vi "ZMQ queue reads.vi"(0 "context in":refnum<class "zmq_context.lvclass">, 1 "Current ZMQ Log":refnum<vi>, 5 "zmq_socket in":refnum<class "zmq_socket.lvclass">, 7 "queue in":refnum<queue>, 9 "Stop":refnum<vi>, 11 "Error in":errorcluster) -> (6 "queue out":refnum<queue>, 10 "ZMQ error out":errorcluster, 15 "Queue error out":errorcluster)   [LabVIEW 2018]
uses:
  <vilib>/addons/zeromq/zmq_socket.lvclass
  Event Sources.ctl
  <vilib>/addons/zeromq/zmq_context.lvclass
  <vilib>/Platform/TimedLoop/XDataNode/timing_clust.ctl
  <vilib>/Platform/TimedLoop/XDataNode/nitl_modes.ctl
  <vilib>/Platform/TimedLoop/XDataNode/wakeup.ctl
  <vilib>/addons/zeromq/poll_type.ctl
  <vilib>/Utility/file.llb/Write Delimited Spreadsheet (string).vi
  <vilib>/addons/zeromq/zmq_poll_scalar.vi
  <vilib>/platform/TimedLoop/XDataNode/XDataNode.xnode
  <vilib>/regexp/Match Regular Expression.xnode
  <vilib>/addons/zeromq/zeromq.lvlib
  <vilib>/Platform/TimedLoop/XDataNode/XDNodeRunTimeDep.lvlib
panel:
  in  "Stop":bool
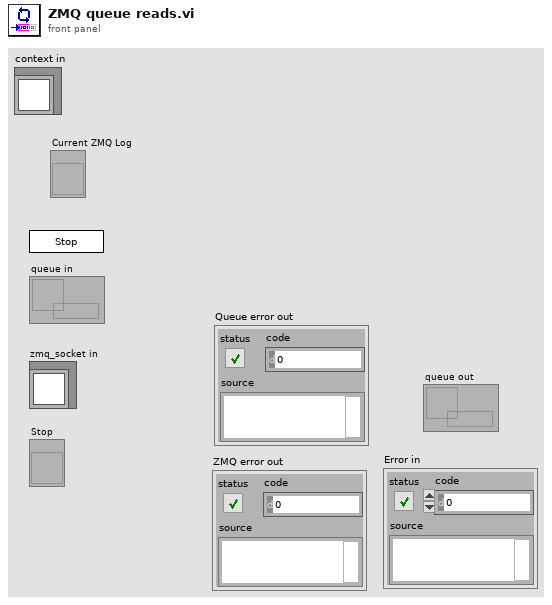
[diagram p1: front panel]
types:
  T1 = typedef "Event Sources.ctl" = enum16{"ZMQ", "INTERNAL", "Check_Errors", "Send_ZMQ_Reply", "Save_PMT_Voltages", "Set_Ramp_Voltage", "Restore PMT Voltages"}
  T2 = typedef "XDNodeRunTimeDep.lvlib/timing_clust.ctl" = cluster{"Expected End [f-1]":u64, "Actual End [f-1]":u64, "Finished Late? [f-1]":bool, "Expected End [i-1]":u64, "Actual End [i-1]":u64, "Finished Late? [i-1]":bool, "Expected Start [i]":u64, "Actual Start [i]":u64, "Expected Start [f]":u64, "Actual Start [f]":u64, "Source Name":string, "Structure Name":string, "Period":i64, "Deadline":i64, "Offset":i64, "Start":i64, "Priority":i32, "Timeout":i32, "Mode":T3, "Wakeup Reason":T4, "Error":errorcluster, "Source Type":string, "Secondary Source Type":string, "Global End Time":u64, "Global Start Time":u64, "Frame Duration":u64, "Iteration Duration":u64, "Assigned CPU":i32, "I/O Scan Engine Mode":u32}
  T3 = typedef "XDNodeRunTimeDep.lvlib/nitl_modes.ctl" = enum32{"No Change", "Process missed periods, maintain original phase", "Discard missed periods, maintain original phase", "Process missed periods, ignore original phase", "Discard missed periods, ignore original phase"}
  T4 = typedef "XDNodeRunTimeDep.lvlib/wakeup.ctl" = enum32{"Normal", "Aborted", "Asynchronous wakeup", "Timing source error", "Timed loop error", "Timeout"}
  T5 = typedef "zeromq.lvlib/poll_type.ctl" = enum16{"None", "In", "Out", "In/Out"}
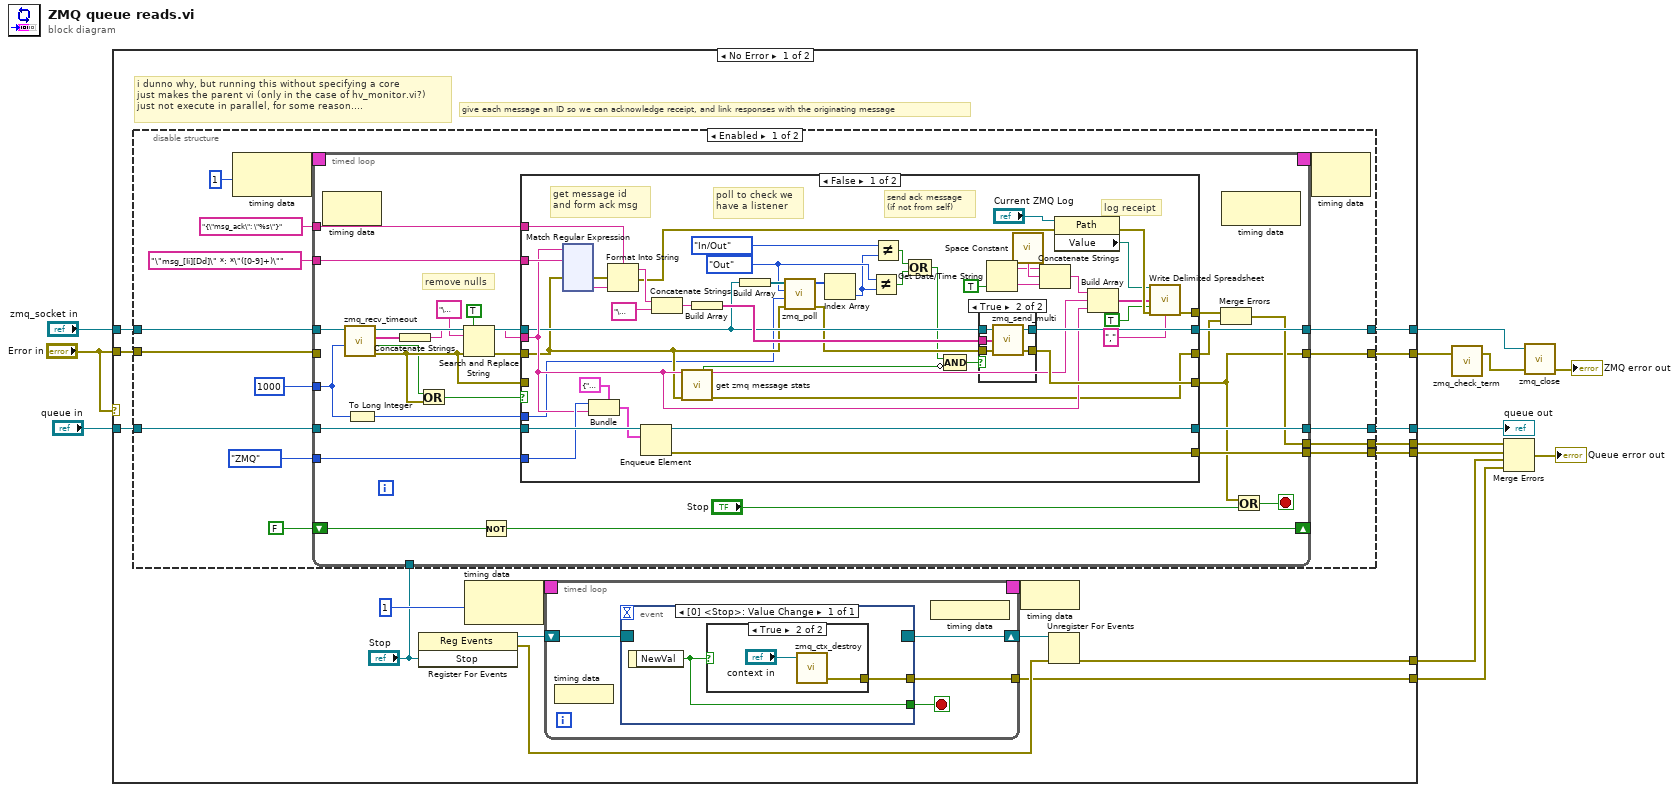
[diagram p0: block diagram]
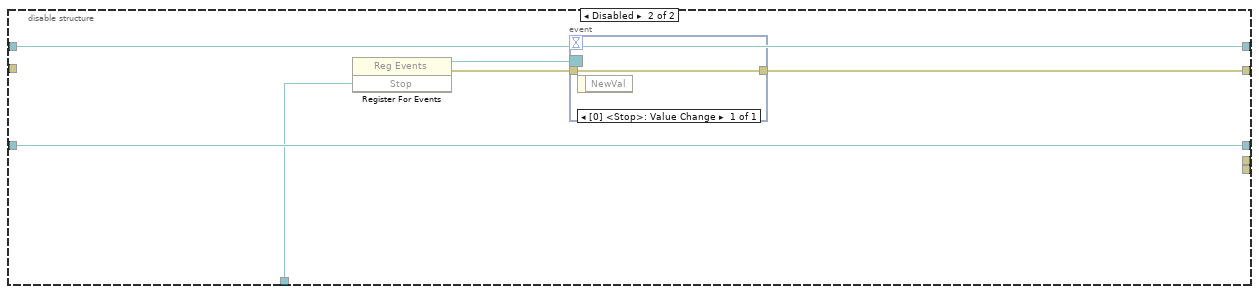
[diagram p4: hidden frame]
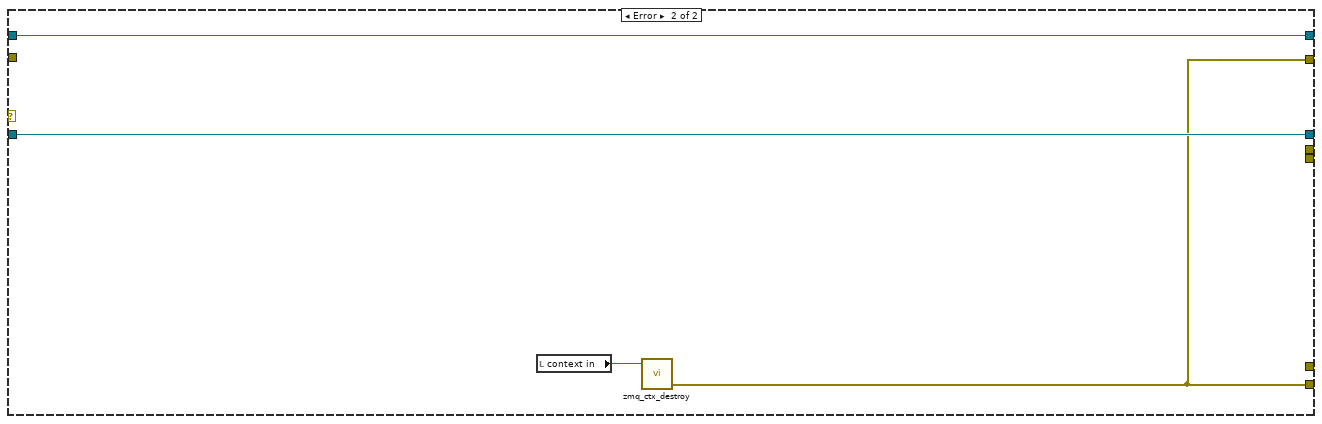
[diagram p6: hidden frame]
diagram:
  n1 = case shown="No Error" "Error in" {
    tunnel: [w28 w276] -> w13
    tunnel: [w25 _] -> w12
    tunnel: [w24 w275] -> w10
    tunnel: [w23 w275] -> w9
    tunnel: [w22 w277] -> w6
    tunnel: [w20 _] -> w5
    tunnel: [w18 _] -> w4
    tunnel: "zmq_socket in" -> [w17 w277]
    tunnel: "queue in" -> [w16 w276]
    tunnel: "Error in" -> [w14 _]
    frame No Error {
      # "i dunno why, but running this without specifying a core\njust makes the parent vi (only in the case of hv_monitor.vi?)\njust not execute in parallel, for some reason...."
      # "give each message an ID so we can acknowledge receipt, and link responses with the originating message"
      n2 = disable-structure shown="Enabled" {
        disable-tunnel: [w43 w258] -> w28
        disable-tunnel: [w38 _] -> w25
        disable-tunnel: [w37 w255] -> w23
        disable-tunnel: [w36 w259] -> w22
        disable-tunnel: [w35 _] -> w20
        disable-tunnel: w17 -> [w31 w259]
        disable-tunnel: w16 -> [w33 w258]
        disable-tunnel: "Stop" -> [_ w256]
        disable-tunnel: w14 -> [w32 _]
        frame Enabled {
          n3 = node-c288(1 ("Processor")) -> (w46:T2)
          n4 = timed-loop {
            tunnel: w31 -> [w49]
            tunnel: [w55] -> w37
            tunnel: w33 -> [w74]
            tunnel: [w72] -> w38
            tunnel: [w68] -> w36
            tunnel: w32 -> [_]
            tunnel: u32 1000 ("timeout (ms)") -> [w48]
            tunnel: [w70] -> w43
            tunnel: "\"msg_[Ii][Dd]\" *: *\"([0-9]+)\"" ("regular expression") -> [w67]
            shift-right: [w65] -> _
            shift-left: FALSE ("Value") -> [w66]
            tunnel: "{\"msg_ack\": \"%s\"}" ("regular expression") -> [w64]
            tunnel: Event_Sources."ZMQ" ("Source") -> [w62]
            tunnel: [w56] -> w35
            timing: w46 -> [_]
            timing-out: [_] -> w45
            stop <- w73 stop-if-true
            # "remove nulls"
            n5 = node-c288() -> ()  [unwired: 1 in, 1 out]
            n6 = call <vilib>:"zmq_recv_timeout.vi"("timeout (ms)"=w48, "socket in"=w49) -> ("error out"=w59:errorcluster, "timeout?"=w53:bool, "parts"=w54:string[], "socket out"=w69:refnum<class "zmq_socket.lvclass">)  [unwired: 2 in]
            n7 = To Long Integer(number=w48) -> (32bit integer=w47:i32)
            n8 = Concatenate Strings(w54) -> (w50:string)
            n9 = Or(x=w53, y=w59) -> (x .or. y?=w63:bool)
            n10 = Search and Replace String(replace all?=TRUE ("replace all? (F)"), input string=w50, search string="\u0000" ("String"), error in=w59) -> (result string=w60:string, error out=w61:errorcluster)  [unwired: 4 in, 2 out]
            n11 = Not(x=w66) -> (.not. x?=w65:bool)
            n12 = case shown="False" w63 {
              tunnel: w74 -> [w122 w247]
              tunnel: [w121 _] -> w72
              tunnel: [w120 w247] -> w70
              tunnel: w69 -> [w90 w249]
              tunnel: [w118 w249] -> w68
              tunnel: [w92 w248] -> w57
              tunnel: w60 -> [w94 _]
              tunnel: w67 -> [w117 _]
              tunnel: w61 -> [w87 w248]
              tunnel: w64 -> [w115 _]
              tunnel: w62 -> [w113 _]
              tunnel: [w96 _] -> w58
              tunnel: [w95 w246] -> w55
              tunnel: w59 -> [_ w246]
              tunnel: w47 -> [w82 _]
              frame False {
                w83 = poll_type."Out" ("poll type")
                # "poll to check we\nhave a listener"
                # "log receipt"
                # "get message id\nand form ack msg"
                # "send ack message\n(if not from self)"
                n13 = xnode "Match Regular Expression"("input string"=w94, "regular expression"=w117, "error in"=w87) -> ("error out"=w116:errorcluster, "submatch 1"=w110:string)  [unwired: 3 in, 4 out]
                n14 = Bundle(cluster=cluster{"Source":T1, "Command":string} {"Source"=enum."ZMQ", "Command"=""} ("output cluster"), "Source"=w113, "Command"=w94) -> (w112:cluster{"Source":T1, "Command":string})
                n15 = Format Into String(format string=w115, error in=w116, w110) -> (resulting string=w114:string, error out=w91:errorcluster)  [unwired: 1 in]
                n16 = Enqueue Element(queue=w122, element=w112) -> (queue out=w120:refnum<queue>, error out=w121:errorcluster)  [unwired: 2 in, 1 out]
                n17 = Concatenate Strings(w114, "\u0000" ("String")) -> (w98:string)
                n18 = call "get zmq message stats.vi"("message"=w94, "error in"=w87) -> ("Self Message"=w85:bool, "msg_id"=w93:string, "error out"=w92:errorcluster)  [unwired: 8 in, 3 out]
                n19 = Build Array(w98) -> (w97:string[])
                n20 = Build Array(w90) -> (w89:refnum<class "zmq_socket.lvclass">[])
                n21 = call-poly <vilib>:"zmq_poll.vi"("error in"=w87, "timeout"=w82, "poll type"=w83, "sockets"=w89) -> ("error out"=w88:errorcluster, "polled events"=w86:T5[])  [unwired: 2 out]
                n22 = Index Array(array=w86) -> (element=w80:T5)  [unwired: 1 in]
                n23 = Not Equal?(x=w83, y=w80) -> (x != y?=w78:bool)
                n24 = Not Equal?(x=poll_type."In/Out" ("poll type"), y=w80) -> (x != y?=w79:bool)
                n25 = Compound Arithmetic op=OR(w79, w78) -> (w77:bool)
                n26 = Compound Arithmetic op=AND(w77, invert w85) -> (w84:bool)
                n27 = case shown="True" w84 {
                  tunnel: w90 -> [w124 w129]
                  tunnel: [w124 w128] -> w118
                  tunnel: w97 -> [_ w127]
                  tunnel: [w123 w126] -> w95
                  tunnel: w88 -> [w123 w125]
                  frame False {
                  }
                  frame True {
                    n28 = call <vilib>:"zmq_send_multi.vi"("error in"=w125, "parts"=w127, "socket in"=w129) -> ("error out"=w126:errorcluster, "socket out"=w128:refnum<class "zmq_socket.lvclass">)  [unwired: 1 in]
                  }
                }
                n29 = Get Date/Time String(want seconds? (F)=TRUE) -> (date string=w99:string, time string=w100:string)  [unwired: 2 in]
                n30 = call <vilib>:"Space Constant.vi"() -> ("String"=w101:string)
                n31 = Concatenate Strings(w99, w101, w100) -> (w103:string)
                n32 = property class="Path"(reference="Current ZMQ Log", error in=w91) -> (error out=w109:errorcluster, "Value"=w108:path)  [unwired: 1 out]
                n33 = Build Array(w103, w93, w94) -> (w104:string[])
                n34 = call-poly <vilib>:"Write Delimited Spreadsheet.vi"("file path (dialog if empty)"=w108, "1D data"=w104, "append to file? (new file:F)"=TRUE ("append to file? (F)"), "error in (no error)"=w109, "delimiter (\\t)"="," ("delimiter (\\t)")) -> ("error out"=w96:errorcluster)  [unwired: 9 in, 1 out]
              }
              frame True {
              }
            }
            n35 = Merge Errors(w58, w57) -> (w56:errorcluster)
            n36 = node-c288() -> ()  [unwired: 1 in, 1 out]
            n37 = Or(x=w55, y="Stop") -> (x .or. y?=w73:bool)
          }
          n38 = node-c288(w45) -> ()  [unwired: 1 out]
        }
        frame Disabled {
          n39 = register-events(w256) -> (reference out=w257:refnum<event-registration>, error out=w254:errorcluster)  [unwired: 2 in]
          n40 = event shown="[0] <Stop>: Value Change" {
            selector: w257 -> [_]
            dyn-events: _ -> [_]
            timeout: _ -> [_]
            tunnel: [w260] -> w255
            tunnel: w254 -> [w260]
            event Value Change {
              n41 = event-data() -> ()  [unwired: 1 in, 1 out]
            }
          }
        }
      }
      n42 = register-events("Stop") -> (reference out=w21:refnum<event-registration>, error out=w26:errorcluster)  [unwired: 2 in]
      n43 = node-c288(1 ("Processor")) -> (w30:T2)
      n44 = timed-loop {
        tunnel: [w262] -> w24
        shift-right: [w263] -> w27
        shift-left: w21 -> [w264]
        timing: w30 -> [_]
        timing-out: [_] -> w29
        stop <- w261 stop-if-true
        n45 = node-c288() -> ()  [unwired: 1 in]
        n46 = event shown="[0] <Stop>: Value Change" {
          selector: w264 -> [_]
          dyn-events: [_] -> w263
          timeout: _ -> [_]
          tunnel: [w268] -> w262
          tunnel: [w267] -> w261
          event Value Change {
            n47 = event-data() -> ("NewVal"=w267:bool)  [unwired: 1 in]
            n48 = case shown="True" w267 {
              tunnel: [_ w269] -> w268
              frame False {
              }
              frame True {
                n49 = call <vilib>:"zmq_ctx_destroy.vi"("context in"="context in") -> ("error out"=w269:errorcluster)  [unwired: 4 in]
              }
            }
          }
        }
        n50 = node-c288() -> ()  [unwired: 1 out]
      }
      n51 = node-c288(w29) -> ()
      n52 = Unregister For Events(event registration refnum=w27, error in=w26) -> (error out=w18:errorcluster)
    }
    frame Error {
      n53 = local read "context in"() -> (w278:refnum<class "zmq_context.lvclass">)
      n54 = call <vilib>:"zmq_ctx_destroy.vi"("context in"=w278) -> ("error out"=w275:errorcluster)  [unwired: 4 in]
    }
  }
  "queue out" <- w13
  n55 = call <vilib>:"zmq_check_term.vi"("error in"=w9) -> ("error out"=w8:errorcluster)  [unwired: 1 in, 1 out]
  n56 = Merge Errors(w5, w12, w4, w10) -> (→"Queue error out":errorcluster)
  n57 = call <vilib>:"zmq_close.vi"("error in"=w8, "socket"=w6) -> ("error out"=→"ZMQ error out":errorcluster)  [unwired: 3 in]
